vi "Empty Block Diagram.vi"(8 "error in (no error)":errorcluster, 11 "VI in":refnum<vi>) -> (0 "error out":errorcluster, 3 "reference out":refnum<vi>)   [LabVIEW 2020, in "Mock Class Generator.lvclass"]
uses:
  Mock Class Generator.lvclass
  <vilib>/Utility/traverseref.llb/TRef TravTarget.ctl
  <vilib>/Utility/miscctls.llb/LVPositionTypeDef.ctl
  <vilib>/Utility/traverseref.llb/VI Scripting - Traverse.lvlib
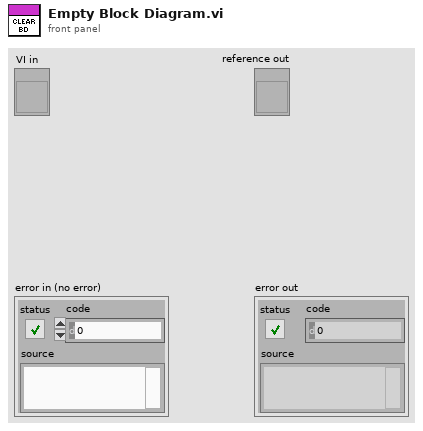
[diagram p1: front panel]
types:
  T1 = typedef "TRef TravTarget.ctl" = enum16{"FP", "BD", "Other"}
  T2 = typedef "LVPositionTypeDef.ctl" = cluster{"Left":i32, "Top":i32}
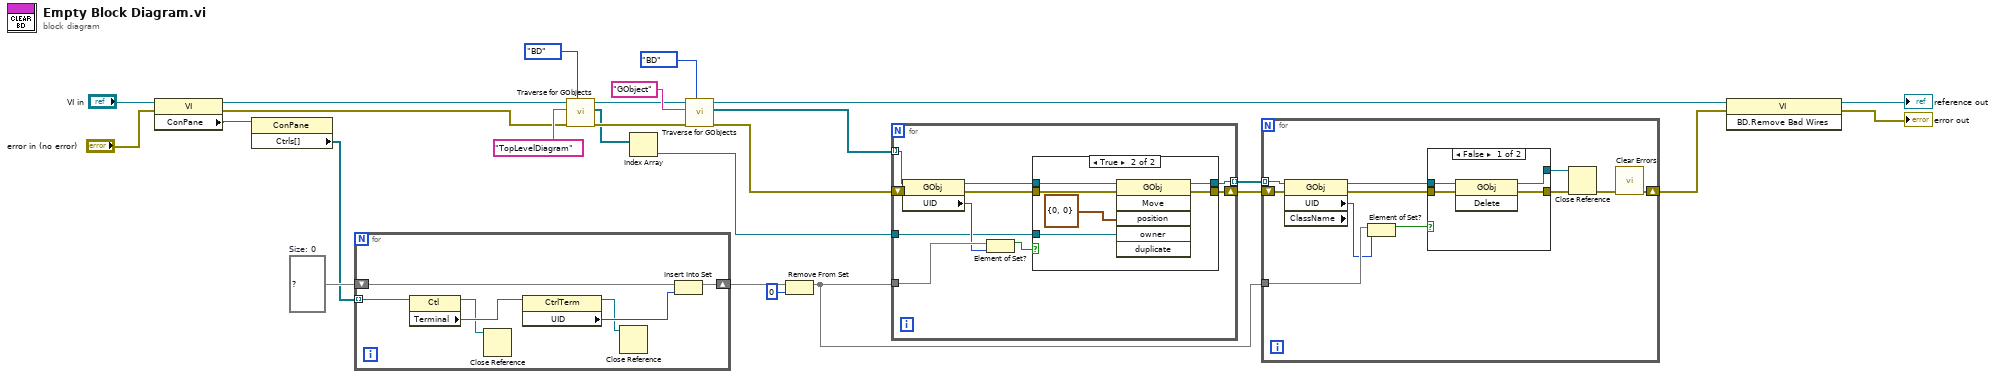
[diagram p0: block diagram]
diagram:
  w19 = set{i32} {}  # Size: 0
  n1 = property class="VI"(reference="VI in", error in="error in (no error)") -> (reference out=w9:refnum<vi>, error out=w7:errorcluster, "ConPane"=w20:refnum<vi>)
  n2 = property class="ConPane"(reference=w20) -> ("Ctrls[]"=w18:refnum<vi>[])  [unwired: 1 in, 2 out]
  n3 = for {
    shift-right: [w31] -> w13
    shift-left: w19 -> [w33]
    tunnel: w18 -> [w32] mode=indexing
    n4 = property class="Ctl"(reference=w32) -> (reference out=w27:refnum<vi>, "Terminal"=w28:refnum<vi>)  [unwired: 1 in, 1 out]
    n5 = Close Reference(reference=w27) -> ()  [unwired: 1 in, 1 out]
    n6 = property class="CtrlTerm"(reference=w28) -> (reference out=w29:refnum<vi>, "UID"=w30:i32)  [unwired: 1 in, 1 out]
    n7 = Close Reference(reference=w29) -> ()  [unwired: 1 in, 1 out]
    n8 = Insert Into Set(10:w30, 11:w33) -> (3:w31:set{i32})  [unwired: 1 out]
  }
  n9 = call <vilib>:"Traverse for GObjects.vi"("Traverse Target"=TRef_TravTarget."BD", "error in (no error)"=w7, "Class Name"="TopLevelDiagram", "VI Refnum"=w9) -> ("error out"=w6:errorcluster, "References"=w4:refnum<vi>[], "dup VI Refnum"=w8:refnum<vi>)  [unwired: 4 in, 1 out]
  n10 = Index Array(array=w4) -> (element=w2:refnum<vi>)  [unwired: 1 in]
  n11 = call <vilib>:"Traverse for GObjects.vi"("Traverse Target"=TRef_TravTarget."BD", "error in (no error)"=w6, "Class Name"="GObject", "VI Refnum"=w8) -> ("error out"=w15:errorcluster, "References"=w23:refnum<vi>[], "dup VI Refnum"=w16:refnum<vi>)  [unwired: 4 in, 1 out]
  n12 = Remove From Set(10:0 ("element"), 11:w13) -> (3:w12:set{i32})  [unwired: 1 out]
  n13 = for {
    tunnel: w23 -> [w43] mode=indexing
    tunnel: w12 -> [w41]
    shift-right: [w40] -> w3
    shift-left: w15 -> [w42]
    tunnel: w2 -> [w35]
    tunnel: [w34] -> w1 mode=indexing
    n14 = property class="GObj"(reference=w43, error in=w42) -> (reference out=w38:refnum<vi>, error out=w39:errorcluster, "UID"=w37:i32)
    n15 = Element of Set?(10:w37, 11:w41) -> (3:w36:bool)
    n16 = case shown="True" w36 {
      tunnel: [w45 w51] -> w34
      tunnel: [w44 w49] -> w40
      tunnel: w39 -> [w44 w48]
      tunnel: w38 -> [w45 w47]
      tunnel: w35 -> [_ w46]
      frame False {
      }
      frame True {
        n17 = invoke class="GObj" method="Move"(reference=w47, error in=w48, "position"=T2 {"Left"=0, "Top"=0}, "owner"=w46) -> (reference out=w51:refnum<vi>, error out=w49:errorcluster)  [unwired: 2 in, 4 out]
      }
    }
  }
  n18 = for {
    tunnel: w12 -> [w61]
    shift-right: [w62] -> w14
    shift-left: w3 -> [w54]
    tunnel: w1 -> [w53] mode=indexing
    n19 = property class="GObj" props=["UID", "ClassName"](reference=w53, error in=w54) -> (reference out=w56:refnum<vi>, error out=w57:errorcluster, "UID"=w55:i32)  [unwired: 1 out]
    n20 = Element of Set?(10:w55, 11:w61) -> (3:w52:bool)
    n21 = case shown="False" w52 {
      tunnel: [w66 w67] -> w60
      tunnel: [w65 w68] -> w58
      tunnel: w57 -> [w64 w67]
      tunnel: w56 -> [w63 w68]
      frame False {
        n22 = invoke class="GObj" method="Delete"(reference=w63, error in=w64) -> (reference out=w65:refnum<vi>, error out=w66:errorcluster)  [unwired: 1 in, 1 out]
      }
      frame True {
      }
    }
    n23 = Close Reference(reference=w58, error in (no error)=w60) -> (error out=w59:errorcluster)
    n24 = call <vilib>:"Clear Errors.vi"("error in (no error)"=w59) -> ("error out"=w62:errorcluster)  [unwired: 5 in, 1 out]
  }
  n25 = invoke class="VI" method="BD.Remove Bad Wires"(reference=w16, error in=w14) -> (reference out=→"reference out":refnum<vi>, error out=→"error out":errorcluster)  [unwired: 1 in, 1 out]
